vi "voltage_divider1.vi"() -> ()   [LabVIEW 2017]
panel:
  in  "vi":dbl
  out "vo":dbl
  in  "R2":dbl
  in  "R1":dbl
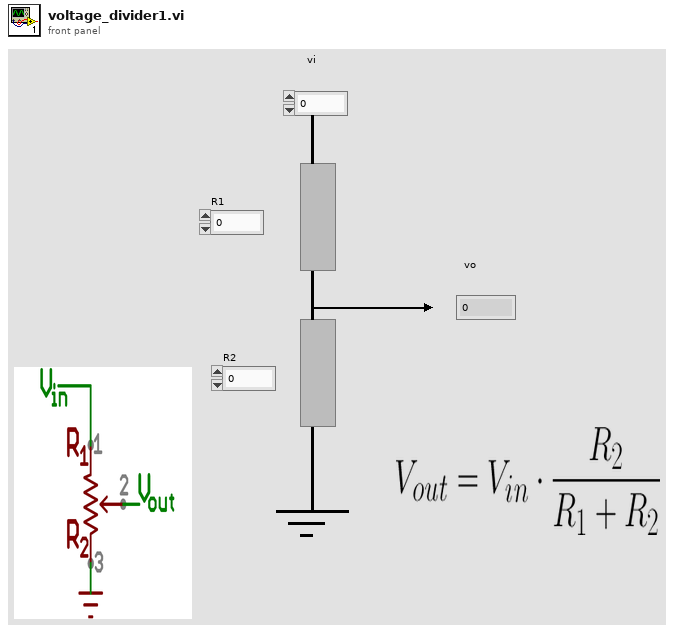
[diagram p1: front panel]
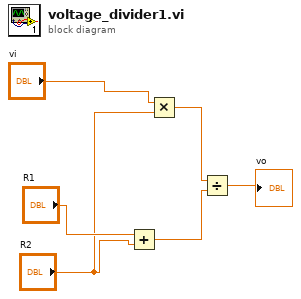
[diagram p0: block diagram]
diagram:
  n1 = Add(x="R1", y="R2") -> (x+y=w2:dbl)
  n2 = Multiply(x="vi", y="R2") -> (x*y=w3:dbl)
  n3 = Divide(x=w3, y=w2) -> (x/y=→"vo":dbl)
